vi "write data files.vi"(8 "error in":errorcluster, 9 "file basename":string, 10 "output folder":path, 11 "WaveformGraph in":refnum<vi>) -> (0 "error out":errorcluster)   [LabVIEW 2020]
uses:
  <vilib>/Utility/file.llb/Write Delimited Spreadsheet (DBL).vi
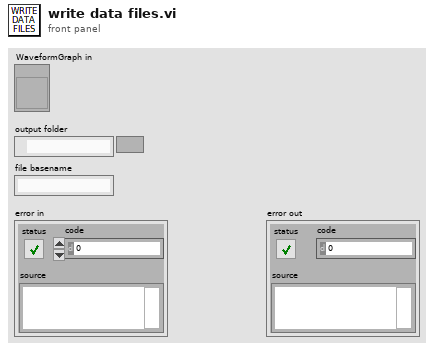
[diagram p1: front panel]
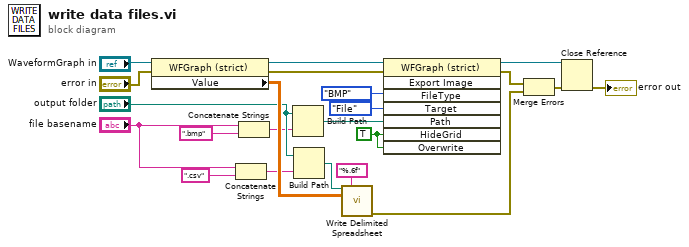
[diagram p0: block diagram]
diagram:
  w17 = TRUE ("Always Overwrite")
  n1 = property class="WFGraph (strict)"(reference="WaveformGraph in", error in="error in") -> (reference out=w11:refnum<vi>, error out=w21:errorcluster, "Value"=w20:dbl[][])
  n2 = Concatenate Strings("file basename", ".csv" ("string")) -> (w6:string)
  n3 = Concatenate Strings("file basename", ".bmp" ("string")) -> (w9:string)
  n4 = Build Path(base path="output folder", name or relative path=w9) -> (appended path=w10:path)
  n5 = Build Path(base path="output folder", name or relative path=w6) -> (appended path=w5:path)
  n6 = call-poly <vilib>:"Write Delimited Spreadsheet.vi"("file path (dialog if empty)"=w5, "format (%.3f)"="%.6f", "2D data"=w20) -> ("error out"=w13:errorcluster)  [unwired: 11 in, 1 out]
  n7 = invoke on="Invoke Node" class="WFGraph (strict)" method="Export Image"(reference=w11, error in=w21, "FileType"=enum32{"BMP", "EPS", "EMF", "PICT"}."BMP" ("File Type"), "Target"=enum32{"File", "Clipboard"}."File", "Path"=w10, "HideGrid"=w17, "Overwrite"=w17) -> (reference out=w14:refnum<vi>, error out=w12:errorcluster)  [unwired: 1 in, 6 out]
  n8 = Merge Errors(w12, w13) -> (w15:errorcluster)
  n9 = Close Reference(reference=w14, error in (no error)=w15) -> (error out=→"error out":errorcluster)
